vi "Odometria2.vi"(6 "left motor ccw velocity (rad/s)":dbl, 9 "Arrastrado":dbl[](array[numeric]), 10 "Zigma":dbl[](array[numeric]), 11 "right motor ccw velocity (rad/s)":dbl) -> ()   [LabVIEW 2011]
uses:
  <vilib>/Analysis/_algsub.llb/Real PseudoInverse Matrix.vi
  <vilib>/Analysis/baseanly.llb/A x Vector.vi
  <vilib>/Analysis/Matrix/Numeric/Conversions/Array To Matrix - RA.vi
  <vilib>/Analysis/baseanly.llb/Real Inverse Matrix.vi
  <vilib>/Analysis/NI_AALPro.lvlib
  <vilib>/Analysis/NI_AALBase.lvlib
  <vilib>/Analysis/Matrix/NI_Matrix.lvlib
panel:
  out "Array out":dbl[](array[numeric])
  out "Arrastrad_out":dbl[](array[numeric])
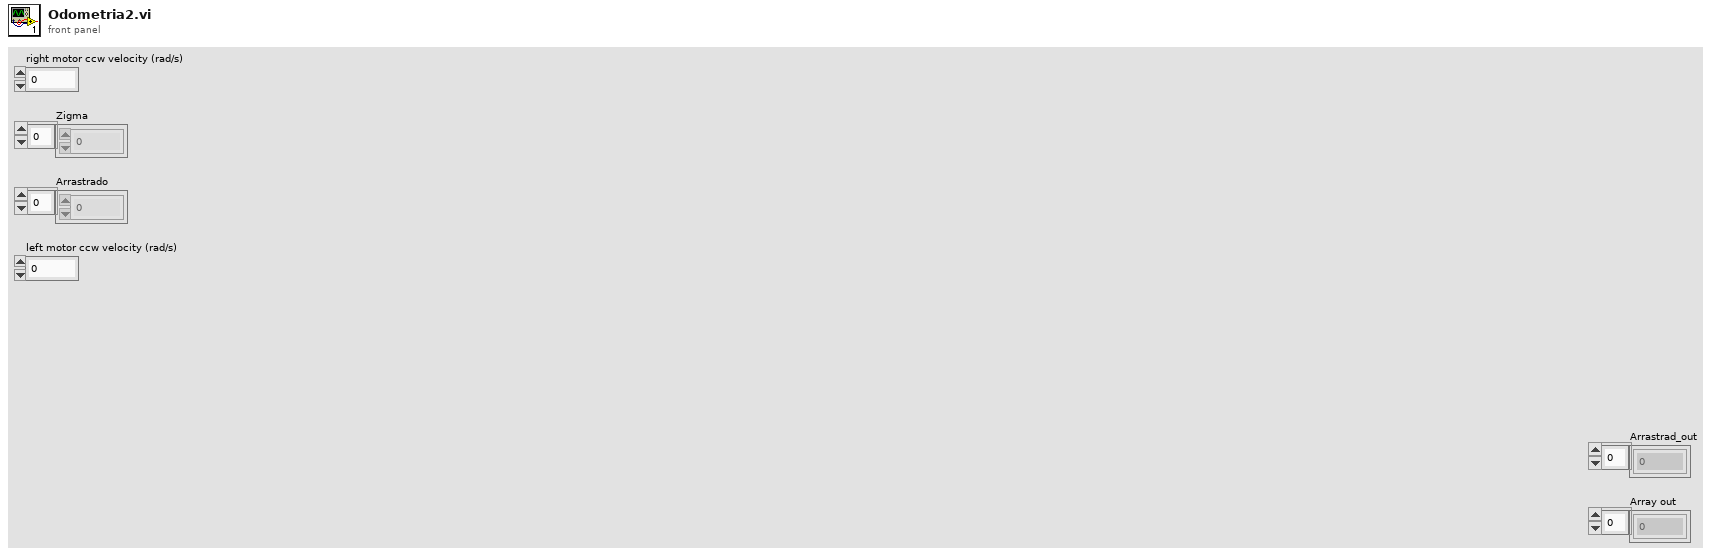
[diagram p1: front panel]
types:
  T1 = typedef "NI_Matrix.lvlib/RealMatrix.ctl" = dbl[][]
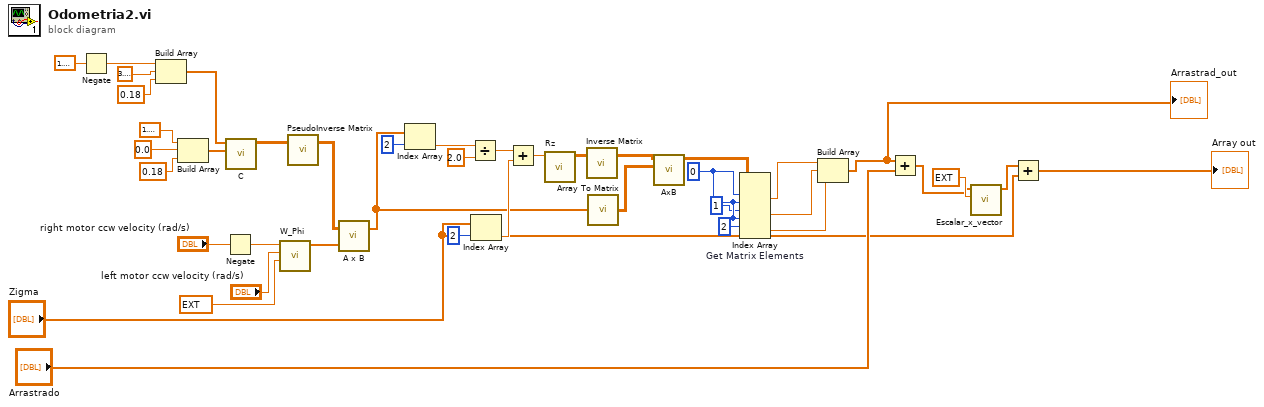
[diagram p0: block diagram]
diagram:
  w7 = 0 ("index (row)")
  n1 = Negate(x=1.5707963267948966) -> (-x=w36:dbl)
  n2 = Build Array(w36, 3.141592653589793, 0.18) -> (w33:dbl[])
  n3 = Build Array(1.5707963267948966, 0.0, 0.18) -> (w32:dbl[])
  n4 = Negate(x="right motor ccw velocity (rad/s)") -> (-x=w26:dbl)
  n5 = call "C.vi"("Llanta 2"=w32, "Llanta 1"=w33) -> ("Matrix Transpose"=w24:T1)  [unwired: 9 in]
  n6 = call "W_Phi.vi"("Radio"=ext 0.025 ("Numeric"), "left motor ccw velocity (rad/s)"="left motor ccw velocity (rad/s)", "right motor ccw velocity (rad/s)"=w26) -> ("Array out"=w22:ext[])  [unwired: 8 in]
  n7 = call-poly <vilib>:"PseudoInverse Matrix.vi"("Input Matrix"=w24) -> ("PseudoInverse Matrix"=w23:T1)  [unwired: 1 in, 1 out]
  n8 = call-poly <vilib>:"A x B.vi"("Vector"=w22, "A"=w23) -> ("A x Vector"=w12:dbl[])  [unwired: 1 out]
  n9 = Index Array(array=w12, index=2) -> (element=w19:dbl)
  n10 = Divide(x=w19, y=2.0) -> (x/y=w17:dbl)
  n11 = Index Array(array="Zigma", index=2) -> (element=w16:dbl)
  n12 = Add(x=w17, y=w16) -> (x+y=w15:dbl)
  n13 = call "Rz.vi"("theta"=w15) -> ("RotacionalZ"=w14:T1)  [unwired: 10 in]
  n14 = call-poly <vilib>:"Inverse Matrix.vi"("Input Matrix"=w14) -> ("Inverse Matrix"=w10:T1)  [unwired: 1 in, 1 out]
  n15 = call-poly <vilib>:"Array To Matrix.vi"("Real 1D Array"=w12) -> ("Real Matrix (Column Vector)"=w11:T1)
  n16 = call "AxB.vi"("B"=w11, "A"=w10) -> ("AxB"=w8:T1)  [unwired: 9 in]
  n17 = Index Array "Get Matrix Elements"(array=w8, index (row) #1=w7, index (col) #1=w7, index (row) #2=1 ("index (row)"), index (col) #2=w7, index (row) #3=2 ("index (row)"), index (col) #3=w7) -> (element #1=w9:dbl, element #2=w4:dbl, element #3=w3:dbl)
  n18 = Build Array(w9, w4, w3) -> (w2:dbl[])
  "Arrastrad_out" <- w2
  n19 = Add(x=w2, y="Arrastrado") -> (x+y=w38:dbl[])
  n20 = call "Escalar_x_vector.vi"("Numeric"=ext 0.01, "Array in"=w38) -> ("Array out"=w39:ext[])  [unwired: 9 in]
  n21 = Add(x=w39, y="Zigma") -> (x+y=→"Array out":ext[])
